vi "Main.vi"(11 "Module Admin":refnum<class "Delacor_lib_QMH_Cloneable Module Admin.lvclass">) -> ()   [LabVIEW 2025, in "Power Supply.lvlib"]
doc: "This template is based off of the Queued Message Handler design pattern and the Queued Message Handler project template that ships with LabVIEW.\n\nThe main difference is that the queue is private to this module and communication between modules is performed via Broadcast and Request events.\n\nRequest events are wrapped in public API methods and are handled in the Event Handling Loop (EHL) of this VI. Any module can register for Broadcast events sent by this module. The EHL generates messages based on user interface actions.\n\nThe Message Handling Loop (MHL) processes messages generated by the EHL, or by other messages. The messages are string values, so new messages can be added easily to the Message Cases case structure in the MHL. Each message cluster can also provide an optional value for Message Data, which is a variant that can be converted to whatever message-specific data is required.\n_____\nBased on DQMH Dev Tools: Project Template 7.1.2.1547."
uses:
  Power Supply.lvlib
  <vilib>/Delacor/Delacor QMH/Libraries/Message Queue_class/Delacor_lib_QMH_Message Queue.lvclass/Delacor_lib_QMH_Message Queue.ctl
  <vilib>/Delacor/Delacor QMH/Libraries/Cloneable Module Admin_class/Delacor_lib_QMH_Cloneable Module Admin.lvclass/Delacor_lib_QMH_Cloneable Module Admin.ctl
  <vilib>/Delacor/Delacor QMH/Libraries/Module Admin_class/Delacor_lib_QMH_Module Admin.lvclass/Delacor_lib_QMH_Module Admin.ctl
  <vilib>/Delacor/Delacor QMH/Libraries/Message Queue_class/Delacor_lib_QMH_Message Queue.lvclass
  Module Data--cluster.ctl
  <vilib>/Utility/miscctls.llb/LVPointTypeDef.ctl
  <vilib>/Delacor/Delacor QMH/Libraries/Message Queue_class/Delacor_lib_QMH_Enqueue Message (Single).vi
  Stop Argument--cluster.ctl
  <vilib>/Delacor/Delacor QMH/Libraries/Cloneable Module Admin_class/Delacor_lib_QMH_Cloneable Module Admin.lvclass
  select child (Reply Payload)--cluster.ctl
  Classes/hardware-selection.ctl
  select child Argument--cluster.ctl
  Classes/generic-power-supply/generic-power-supply.lvclass
  Classes/PSP-603/PSP-603.lvclass
  read config (Reply Payload)--cluster.ctl
  read config Argument--cluster.ctl
  init device (Reply Payload)--cluster.ctl
  init device Argument--cluster.ctl
  close (Reply Payload)--cluster.ctl
  close Argument--cluster.ctl
  output (Reply Payload)--cluster.ctl
  output Argument--cluster.ctl
  set voltage (Reply Payload)--cluster.ctl
  set voltage Argument--cluster.ctl
  set current (Reply Payload)--cluster.ctl
  set current Argument--cluster.ctl
  Controls/Numeric Current.ctl
  read current (Reply Payload)--cluster.ctl
  read current Argument--cluster.ctl
  Controls/Numeric Voltage.ctl
  read voltage (Reply Payload)--cluster.ctl
  read voltage Argument--cluster.ctl
  C:/Users/grove/Desktop/LabVIEW/Git/dqmh-lvoop-template/Libraries/Power Supply/Classes/generic-power-supply/generic-power-supply.lvclass
  C:/Users/grove/Desktop/LabVIEW/Git/dqmh-lvoop-template/Libraries/Power Supply/Classes/PSP-603/PSP-603.lvclass
panel:
  out "error out":errorcluster
  out "Status":string
  in  "Simulate EHL Error":bool
  in  "Simulate MHL Error":bool
  # "Other processes communicate with this Module via its Public API (wrappers for its Request Events).\n\nThis Module communicates with other processes via its Broadcast Events.\nAny process that wants to receive these messages can register for this module's Broadcast events."
  # "This template is for the DQMH framework. See the block diagram for more information on how to use this template."
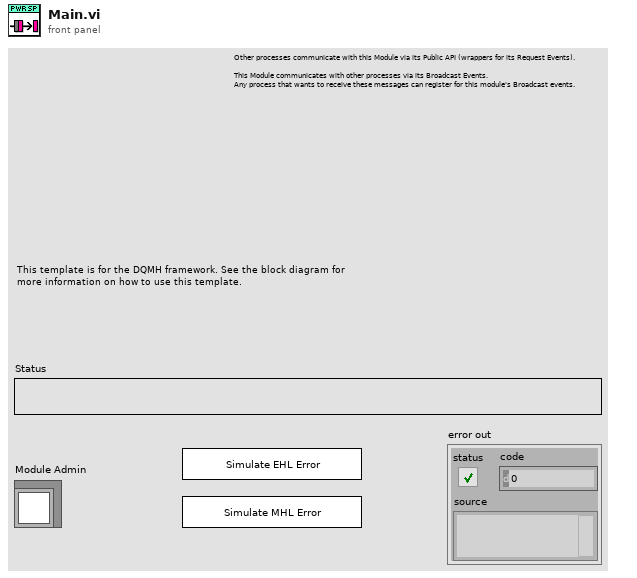
[diagram p1: front panel]
types:
  T1 = typedef "Power Supply.lvlib/Request Events--cluster.ctl" = cluster{"Stop Module":refnum<user-event>, "Show Panel":refnum<user-event>, "Hide Panel":refnum<user-event>, "Show Diagram":refnum<user-event>, "Get Module Execution Status":refnum<user-event>, "select child":refnum<user-event>, "read config":refnum<user-event>, "init device":refnum<user-event>, "close":refnum<user-event>, "output":refnum<user-event>, "set voltage":refnum<user-event>, "set current":refnum<user-event>, "read current":refnum<user-event>, "read voltage":refnum<user-event>}
  T2 = typedef "Power Supply.lvlib/Module Data--cluster.ctl" = cluster{"Status":string, "Power Supply Object":refnum<class "generic-power-supply.lvclass">}
  T3 = enum32{"invalid lock state", "Not Locked", "Locked (No Password)", "Password-protected"}
  T4 = typedef "Power Supply.lvlib/Stop Argument--cluster.ctl" = cluster{"Module ID":i32, "Origin":string, "Exit via Stop Module Req?":bool, "Wait for Module to stop?":bool}
  T5 = typedef "Power Supply.lvlib/select child Argument--cluster.ctl" = cluster{"Module ID":i32, "Enum":T6, "Wait Notifier":refnum<notifier>, "wait for reply":bool}
  T6 = typedef "hardware-selection.ctl" = enum16{"Parent", "Simulation", "PSP-603"}
  T7 = typedef "Power Supply.lvlib/read config Argument--cluster.ctl" = cluster{"Module ID":i32, "config json file":path, "Wait Notifier":refnum<notifier>, "wait for reply":bool}
  T8 = typedef "Power Supply.lvlib/init device Argument--cluster.ctl" = cluster{"Module ID":i32, "Variant":variant, "Wait Notifier":refnum<notifier>, "wait for reply":bool}
  T9 = typedef "Power Supply.lvlib/close Argument--cluster.ctl" = cluster{"Module ID":i32, "Wait Notifier":refnum<notifier>, "wait for reply":bool}
  T10 = typedef "Power Supply.lvlib/output Argument--cluster.ctl" = cluster{"Module ID":i32, "Output On/Off":bool, "Wait Notifier":refnum<notifier>, "wait for reply":bool}
  T11 = typedef "Power Supply.lvlib/set voltage Argument--cluster.ctl" = cluster{"Module ID":i32, "Output Voltage":dbl, "Wait Notifier":refnum<notifier>, "wait for reply":bool}
  T12 = typedef "Power Supply.lvlib/set current Argument--cluster.ctl" = cluster{"Module ID":i32, "Output Current":dbl, "Wait Notifier":refnum<notifier>, "wait for reply":bool}
  T13 = typedef "Power Supply.lvlib/read current Argument--cluster.ctl" = cluster{"Module ID":i32, "Wait Notifier":refnum<notifier>, "wait for reply":bool}
  T14 = typedef "Power Supply.lvlib/read voltage Argument--cluster.ctl" = cluster{"Module ID":i32, "Wait Notifier":refnum<notifier>, "wait for reply":bool}
  T15 = typedef "LVPointTypeDef.ctl" = cluster{"Horizontal":i16, "Vertical":i16}
  T16 = enum32{"Invalid", "Standard", "Closed", "Hidden", "Minimized", "Maximized"}
  T17 = typedef "Power Supply.lvlib/select child (Reply Payload)--cluster.ctl" = cluster{"Module ID":i32, "error":errorcluster}
  T18 = typedef "Power Supply.lvlib/read config (Reply Payload)--cluster.ctl" = cluster{"Module ID":i32, "error":errorcluster}
  T19 = typedef "Power Supply.lvlib/init device (Reply Payload)--cluster.ctl" = cluster{"Module ID":i32, "error":errorcluster}
  T20 = typedef "Power Supply.lvlib/close (Reply Payload)--cluster.ctl" = cluster{"Module ID":i32, "error":errorcluster}
  T21 = typedef "Power Supply.lvlib/output (Reply Payload)--cluster.ctl" = cluster{"Module ID":i32, "error":errorcluster}
  T22 = typedef "Power Supply.lvlib/set voltage (Reply Payload)--cluster.ctl" = cluster{"Module ID":i32, "error":errorcluster}
  T23 = typedef "Power Supply.lvlib/set current (Reply Payload)--cluster.ctl" = cluster{"Module ID":i32, "error":errorcluster}
  T24 = typedef "Power Supply.lvlib/read current (Reply Payload)--cluster.ctl" = cluster{"Module ID":i32, "Amps":T25, "error":errorcluster}
  T25 = typedef "Numeric Current.ctl" = dbl
  T26 = typedef "Power Supply.lvlib/read voltage (Reply Payload)--cluster.ctl" = cluster{"Module ID":i32, "Volts":T27, "error":errorcluster}
  T27 = typedef "Numeric Voltage.ctl" = dbl
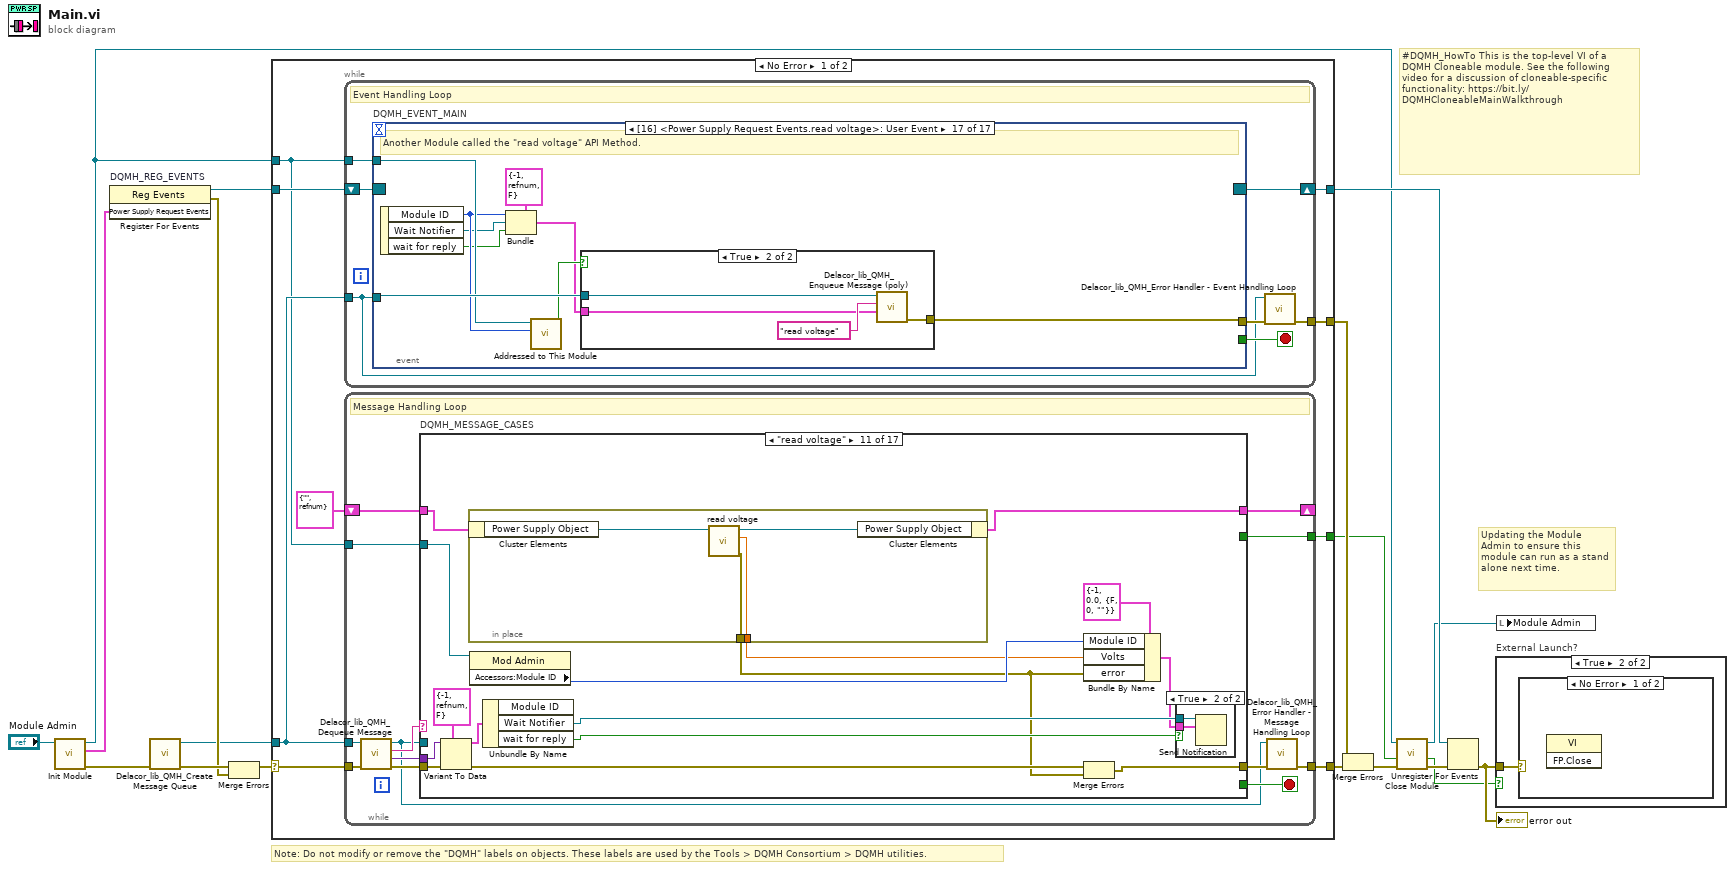
[diagram p0: block diagram]
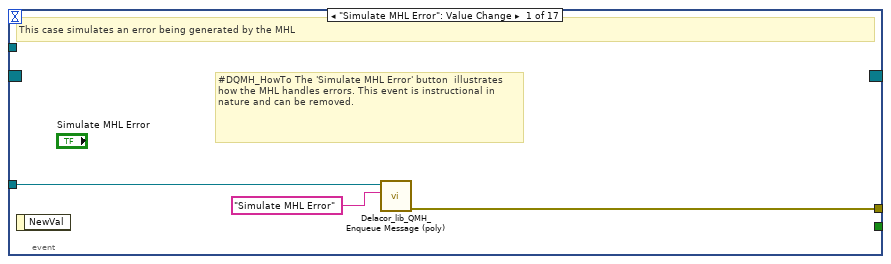
[diagram p2: hidden frame]
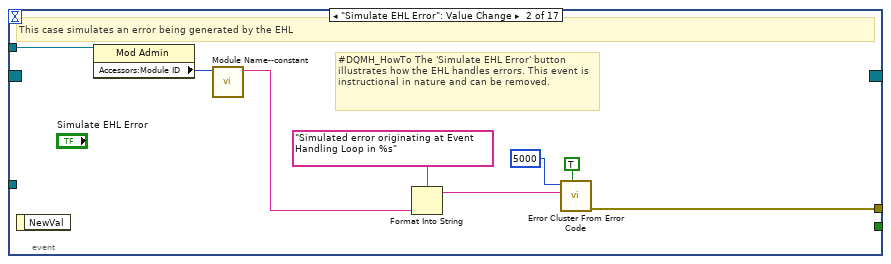
[diagram p3: hidden frame]
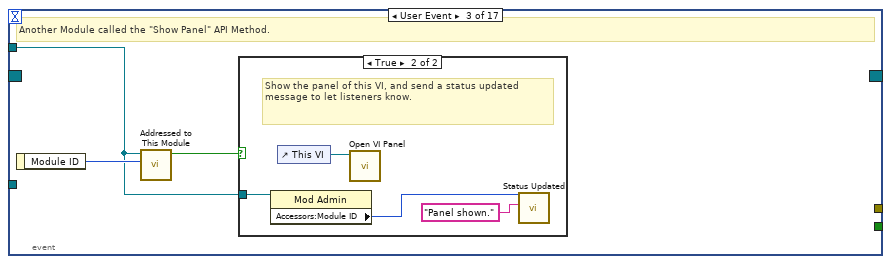
[diagram p4: hidden frame]
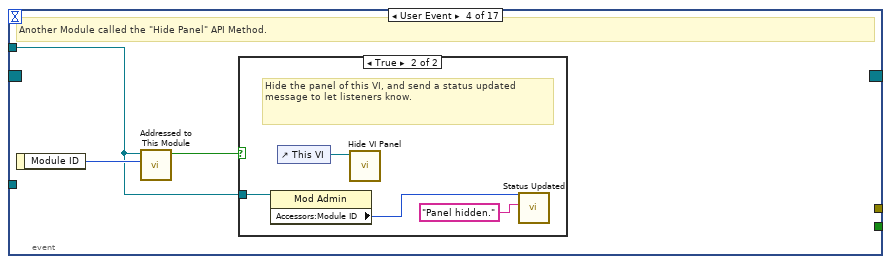
[diagram p6: hidden frame]
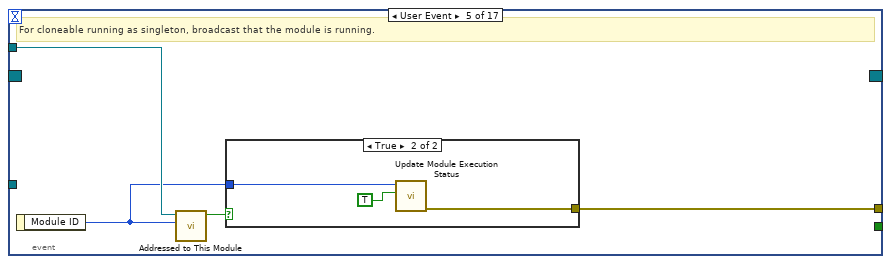
[diagram p8: hidden frame]
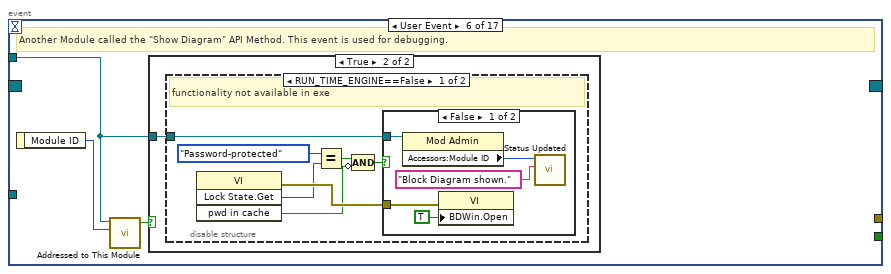
[diagram p10: hidden frame]
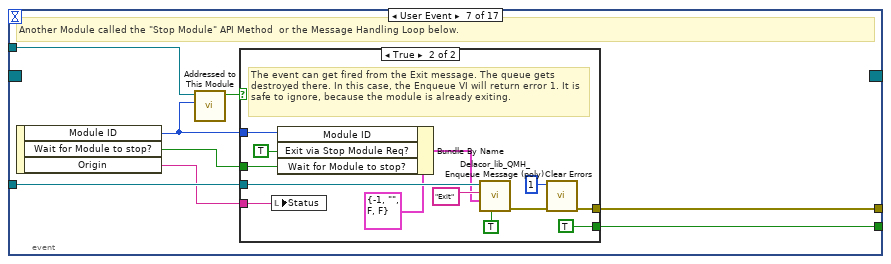
[diagram p14: hidden frame]
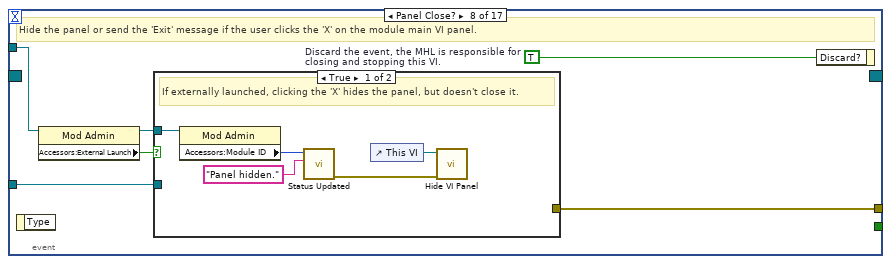
[diagram p16: hidden frame]
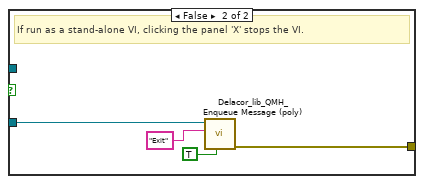
[diagram p17: hidden frame]
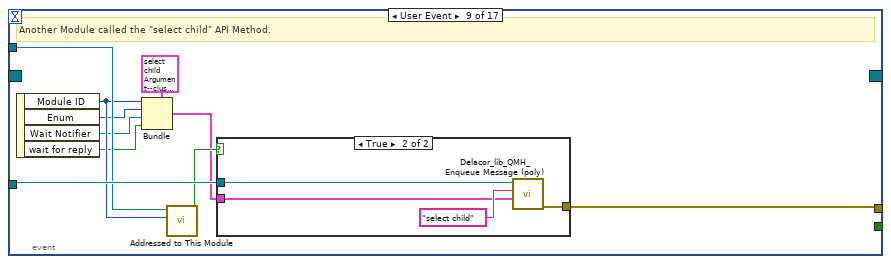
[diagram p18: hidden frame]
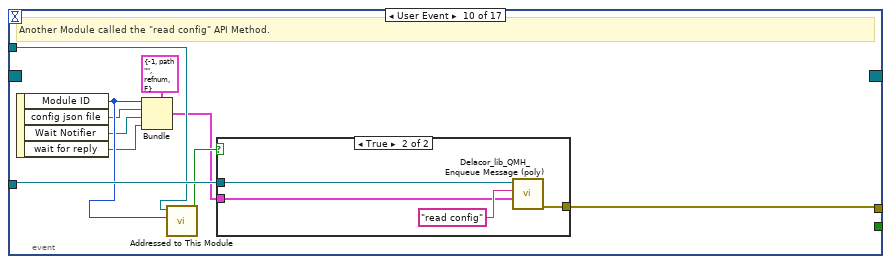
[diagram p20: hidden frame]
diagram:
  # "#DQMH_HowTo This is the top-level VI of a DQMH Cloneable module. See the following video for a discussion of cloneable-specific functionality: https://bit.ly/DQMHCloneableMainWalkthrough"
  # "Note: Do not modify or remove the \"DQMH\" labels on objects. These labels are used by the Tools > DQMH Consortium > DQMH utilities."
  # "Updating the Module Admin to ensure this module can run as a stand alone next time."
  n1 = call "Init Module.vi"("Cloneable Module Admin in"="Module Admin") -> ("error out"=w15:errorcluster, "Power Supply Request Events"=w7:T1, "Cloneable Module Admin out"=w4:refnum<class "Delacor_lib_QMH_Cloneable Module Admin.lvclass">)  [unwired: 8 in]
  n2 = register-events "DQMH_REG_EVENTS"(w7) -> (reference out=w8:refnum<event-registration>, error out=w10:errorcluster)  [unwired: 2 in]
  n3 = call <vilib>:"Delacor_lib_QMH_Create Message Queue.vi"("error in"=w15) -> ("error out"=w12:errorcluster, "Message Queue"=w6:refnum<class "Delacor_lib_QMH_Message Queue.lvclass">)  [unwired: 9 in]
  n4 = Merge Errors(w12, w10) -> (w11:errorcluster)
  n5 = case shown="No Error" w11 {
    selector: w11 -> [w25 w547]
    tunnel: [w27 w546] -> w16
    tunnel: [w24 w545] -> w9
    tunnel: w8 -> [w22 w545]
    tunnel: w6 -> [w21 w538]
    tunnel: [w26 _] -> w17
    tunnel: w4 -> [w20 w541]
    tunnel: [w19 _] -> w2
    frame No Error {
      n6 = while {
        tunnel: w21 -> [w28]
        shift-right: [w31] -> w24
        shift-left: w22 -> [w32]
        tunnel: [w33] -> w26
        tunnel: w20 -> [w29]
        stop <- w30 stop-if-true
        # "Event Handling Loop"
        n7 = event "DQMH_EVENT_MAIN" shown="[16] <Power Supply Request Events.read voltage>: User Event" {
          selector: w32 -> [_ _ _ _ _ _ _ _ _ _ _ _ _ _ _ _ _]
          dyn-events: [_ _ _ _ _ _ _ _ _ _ _ _ _ _ _ _ _] -> w31
          timeout: _ -> [_ _ _ _ _ _ _ _ _ _ _ _ _ _ _ _ _]
          tunnel: [_ _ _ _ _ _ w86 _ _ _ _ _ _ _ _ _ _] -> w30
          tunnel: w28 -> [w36 _ _ _ _ _ w89 w106 w128 w142 w156 w169 w183 w197 w211 w224 w237]
          tunnel: [w37 w45 _ _ w63 _ w90 w109 w119 w133 w147 w161 w174 w188 w202 w216 w229] -> w34
          tunnel: w29 -> [_ w44 w46 w53 w61 w67 w88 w107 w126 w140 w154 w167 w181 w195 w209 w222 w235]
          event "Simulate MHL Error": Value Change {
            # "#DQMH_HowTo The 'Simulate MHL Error' button  illustrates how the MHL handles errors. This event is instructional in nature and can be removed."
            # "This case simulates an error being generated by the MHL"
            n8 = event-data() -> ()  [unwired: 1 in, 1 out]
            n9 = call-poly <vilib>:"Delacor_lib_QMH_Enqueue Message (poly).vi"("Message"="Simulate MHL Error", "Message Queue in"=w36) -> ("error out"=w37:errorcluster)  [unwired: 8 in, 1 out]
          }
          event "Simulate EHL Error": Value Change {
            # "#DQMH_HowTo The 'Simulate EHL Error' button  illustrates how the EHL handles errors. This event is instructional in nature and can be removed."
            # "This case simulates an error being generated by the EHL"
            n10 = event-data() -> ()  [unwired: 1 in, 1 out]
            n11 = property on="Property Node" class="Mod Admin"(reference=w44) -> ("Accessors:Module ID"=w43:i32)  [unwired: 1 in, 2 out]
            n12 = call "Module Name--constant.vi"("Module ID"=w43) -> ("Module Name"=w38:string)  [unwired: 10 in]
            n13 = Format Into String(format string="Simulated error originating at Event Handling Loop in %s", w38) -> (resulting string=w41:string)  [unwired: 2 in, 1 out]
            n14 = call <vilib>:"Error Cluster From Error Code.vi"("show call chain? (False)"=TRUE, "error message (\"\")"=w41, "error code (0)"=5000) -> ("error out"=w45:errorcluster)  [unwired: 6 in]
          }
          event User Event {
            # "Another Module called the \"Show Panel\" API Method."
            n15 = event-data() -> ("Module ID"=w47:i32)  [unwired: 1 in]
            n16 = call "Addressed to This Module.vi"("Module ID from Argument"=w47, "Module Admin"=w46) -> ("Addressed to this instance?"=w48:bool)  [unwired: 8 in, 1 out]
            n17 = case shown="True" w48 {
              tunnel: w46 -> [_ w50]
              frame False {
              }
              frame True {
                # "Show the panel of this VI, and send a status updated message to let listeners know."
                n18 = property on="Property Node" class="Mod Admin"(reference=w50) -> ("Accessors:Module ID"=w49:i32)  [unwired: 1 in, 2 out]
                n19 = control-ref of="This VI"() -> (w52:refnum<vi>)
                n20 = call "Open VI Panel.vi"("VI"=w52) -> ()  [unwired: 10 in, 1 out]
                n21 = call "Status Updated.vi"("Status"="Panel shown." ("format string"), "Module ID"=w49) -> ()  [unwired: 9 in, 1 out]
              }
            }
          }
          event User Event {
            # "Another Module called the \"Hide Panel\" API Method."
            n22 = event-data() -> ("Module ID"=w54:i32)  [unwired: 1 in]
            n23 = call "Addressed to This Module.vi"("Module ID from Argument"=w54, "Module Admin"=w53) -> ("Addressed to this instance?"=w55:bool)  [unwired: 8 in, 1 out]
            n24 = case shown="True" w55 {
              tunnel: w53 -> [_ w57]
              frame False {
              }
              frame True {
                # "Hide the panel of this VI, and send a status updated message to let listeners know."
                n25 = property on="Property Node" class="Mod Admin"(reference=w57) -> ("Accessors:Module ID"=w56:i32)  [unwired: 1 in, 2 out]
                n26 = control-ref of="This VI"() -> (w59:refnum<vi>)
                n27 = call "Hide VI Panel.vi"("VI"=w59) -> ()  [unwired: 10 in, 1 out]
                n28 = call "Status Updated.vi"("Status"="Panel hidden." ("format string"), "Module ID"=w56) -> ()  [unwired: 9 in, 1 out]
              }
            }
          }
          event User Event {
            # "For cloneable running as singleton, broadcast that the module is running."
            n29 = event-data() -> ("Module ID"=w60:i32)  [unwired: 1 in]
            n30 = call "Addressed to This Module.vi"("Module ID from Argument"=w60, "Module Admin"=w61) -> ("Addressed to this instance?"=w62:bool)  [unwired: 8 in, 1 out]
            n31 = case shown="True" w62 {
              tunnel: [_ w66] -> w63
              tunnel: w60 -> [_ w65]
              frame False {
              }
              frame True {
                n32 = call "Update Module Execution Status.vi"("Running?"=TRUE, "Module ID"=w65) -> ("error out"=w66:errorcluster)  [unwired: 9 in]
              }
            }
          }
          event User Event {
            # "Another Module called the \"Show Diagram\" API Method. This event is used for debugging."
            n33 = event-data() -> ("Module ID"=w68:i32)  [unwired: 1 in]
            n34 = call "Addressed to This Module.vi"("Module ID from Argument"=w68, "Module Admin"=w67) -> ("Addressed to this instance?"=w69:bool)  [unwired: 8 in, 1 out]
            n35 = case shown="True" w69 {
              tunnel: w67 -> [_ w70]
              frame False {
              }
              frame True {
                n36 = disable-structure shown="RUN_TIME_ENGINE==False" {
                  disable-tunnel: w70 -> [w71 _]
                  frame condition #0 (active) {
                    # "functionality not available in exe"
                    n37 = invoke on="Invoke Node" class="VI" method="Lock State.Get"() -> (error out=w77:errorcluster, "Get Lock State"=w76:T3, "pwd in cache"=w73:bool)  [unwired: 4 in, 1 out]
                    n38 = Equal?(x=T3."Password-protected", y=w76) -> (x = y?=w74:bool)
                    n39 = Compound Arithmetic op=AND(w74, invert w73) -> (w72:bool)
                    n40 = case shown="False" w72 {
                      tunnel: w77 -> [w82 _]
                      tunnel: w71 -> [w79 _]
                      frame False {
                        n41 = property on="Property Node" class="Mod Admin"(reference=w79) -> ("Accessors:Module ID"=w78:i32)  [unwired: 1 in, 2 out]
                        n42 = property on="Property Node" class="VI"(error in=w82, "BDWin.Open"=TRUE ("Block Diagram Window:Open")) -> ()  [unwired: 1 in, 2 out]
                        n43 = call "Status Updated.vi"("Status"="Block Diagram shown." ("format string"), "Module ID"=w78) -> ()  [unwired: 9 in, 1 out]
                      }
                      frame True {
                        # "Password-protected VI, and the password is not in the cache. Do not show the diagram."
                      }
                    }
                  }
                  frame condition #1 {
                  }
                }
              }
            }
          }
          event User Event {
            # "Another Module called the \"Stop Module\" API Method  or the Message Handling Loop below."
            n44 = event-data() -> ("Module ID"=w84:i32, "Wait for Module to stop?"=w85:bool, "Origin"=w83:string)  [unwired: 1 in]
            n45 = call "Addressed to This Module.vi"("Module ID from Argument"=w84, "Module Admin"=w88) -> ("Addressed to this instance?"=w87:bool)  [unwired: 8 in, 1 out]
            n46 = case shown="True" w87 {
              tunnel: [_ w102] -> w90
              tunnel: w89 -> [_ w98]
              tunnel: [_ TRUE] -> w86
              tunnel: w85 -> [_ w93]
              tunnel: w84 -> [_ w95]
              tunnel: w83 -> [_ w91]
              frame False {
              }
              frame True {
                # "The event can get fired from the Exit message. The queue gets destroyed there. In this case, the Enqueue VI will return error 1. It is safe to ignore, because the module is already exiting."
                n47 = local write "Status"(w91) -> ()
                n48 = Bundle By Name(cluster=T4 {"Module ID"=-1, "Origin"="", "Exit via Stop Module Req?"=FALSE, "Wait for Module to stop?"=FALSE} ("Stop Argument"), "Module ID"=w95, "Exit via Stop Module Req?"=TRUE, "Wait for Module to stop?"=w93) -> (w92:T4)
                n49 = call-poly <vilib>:"Delacor_lib_QMH_Enqueue Message (poly).vi"("Priority Message? (F)"=TRUE, "Message Data"=w92, "Message"="Exit", "Message Queue in"=w98) -> ("error out"=w103:errorcluster)  [unwired: 6 in, 1 out]
                n50 = call <vilib>:"Clear Errors.vi"("error in (no error)"=w103, "specific error code to clear (0: all)"=1) -> ("error out"=w102:errorcluster)  [unwired: 4 in, 1 out]
              }
            }
          }
          event Panel Close? {
            w108 = TRUE  # Discard the event, the MHL is responsible for closing and stopping this VI.
            # "Hide the panel or send the 'Exit' message if the user clicks the 'X' on the module main VI panel."
            n51 = event-data() -> ()  [unwired: 1 in, 1 out]
            n52 = property on="Property Node" class="Mod Admin"(reference=w107) -> (reference out=w104:refnum<class "Delacor_lib_QMH_Cloneable Module Admin.lvclass">, "Accessors:External Launch"=w105:bool)  [unwired: 1 in, 1 out]
            n53 = case shown="True" w105 {
              tunnel: w106 -> [_ w117]
              tunnel: [_ w118] -> w109
              tunnel: w104 -> [w112 _]
              frame True {
                # "If externally launched, clicking the 'X' hides the panel, but doesn't close it."
                n54 = property on="Property Node" class="Mod Admin"(reference=w112) -> ("Accessors:Module ID"=w111:i32)  [unwired: 1 in, 2 out]
                n55 = call "Status Updated.vi"("Status"="Panel hidden." ("format string"), "Module ID"=w111) -> ("error out"=w110:errorcluster)  [unwired: 9 in]
                n56 = control-ref of="This VI"() -> (w114:refnum<vi>)
                n57 = call "Hide VI Panel.vi"("error in"=w110, "VI"=w114) -> ()  [unwired: 9 in, 1 out]
              }
              frame False {
                # "If run as a stand-alone VI, clicking the panel 'X' stops the VI."
                n58 = call-poly <vilib>:"Delacor_lib_QMH_Enqueue Message (poly).vi"("Priority Message? (F)"=TRUE, "Message"="Exit", "Message Queue in"=w117) -> ("error out"=w118:errorcluster)  [unwired: 7 in, 1 out]
              }
            }
            n59 = event-data ("Event Filter Node")("Discard?"=w108) -> ()  [unwired: 1 in, 1 out]
          }
          event User Event {
            # "Another Module called the \"select child\" API Method."
            n60 = event-data() -> ("Module ID"=w123:i32, "Enum"=w122:T6, "Wait Notifier"=w121:refnum<notifier>, "wait for reply"=w120:bool)  [unwired: 1 in]
            n61 = Bundle(cluster=T5 {"Module ID"=-1, "Enum"=enum."PSP-603", "Wait Notifier"=refnum, "wait for reply"=FALSE} ("select child Argument"), "Module ID"=w123, "Enum"=w122, "Wait Notifier"=w121, "wait for reply"=w120) -> (w124:T5)
            n62 = call "Addressed to This Module.vi"("Module ID from Argument"=w123, "Module Admin"=w126) -> ("Addressed to this instance?"=w127:bool)  [unwired: 8 in, 1 out]
            n63 = case shown="True" w127 {
              tunnel: w128 -> [_ w132]
              tunnel: w124 -> [_ w130]
              tunnel: [_ w129] -> w119
              frame False {
              }
              frame True {
                n64 = call-poly <vilib>:"Delacor_lib_QMH_Enqueue Message (poly).vi"("Message Data"=w130, "Message"="select child", "Message Queue in"=w132) -> ("error out"=w129:errorcluster)  [unwired: 7 in, 1 out]
              }
            }
          }
          event User Event {
            # "Another Module called the \"read config\" API Method."
            n65 = event-data() -> ("Module ID"=w137:i32, "config json file"=w136:path, "Wait Notifier"=w135:refnum<notifier>, "wait for reply"=w134:bool)  [unwired: 1 in]
            n66 = Bundle(cluster=T7 {"Module ID"=-1, "config json file"=path "", "Wait Notifier"=refnum, "wait for reply"=FALSE} ("read config Argument"), "Module ID"=w137, "config json file"=w136, "Wait Notifier"=w135, "wait for reply"=w134) -> (w138:T7)
            n67 = call "Addressed to This Module.vi"("Module ID from Argument"=w137, "Module Admin"=w140) -> ("Addressed to this instance?"=w141:bool)  [unwired: 8 in, 1 out]
            n68 = case shown="True" w141 {
              tunnel: w142 -> [_ w146]
              tunnel: w138 -> [_ w144]
              tunnel: [_ w143] -> w133
              frame False {
              }
              frame True {
                n69 = call-poly <vilib>:"Delacor_lib_QMH_Enqueue Message (poly).vi"("Message Data"=w144, "Message"="read config", "Message Queue in"=w146) -> ("error out"=w143:errorcluster)  [unwired: 7 in, 1 out]
              }
            }
          }
          event User Event {
            # "Another Module called the \"init device\" API Method."
            n70 = event-data() -> ("Module ID"=w151:i32, "Variant"=w150:variant, "Wait Notifier"=w149:refnum<notifier>, "wait for reply"=w148:bool)  [unwired: 1 in]
            n71 = Bundle(cluster=T8 {"Module ID"=-1, "Variant"=variant, "Wait Notifier"=refnum, "wait for reply"=FALSE} ("init device Argument"), "Module ID"=w151, "Variant"=w150, "Wait Notifier"=w149, "wait for reply"=w148) -> (w152:T8)
            n72 = call "Addressed to This Module.vi"("Module ID from Argument"=w151, "Module Admin"=w154) -> ("Addressed to this instance?"=w155:bool)  [unwired: 8 in, 1 out]
            n73 = case shown="True" w155 {
              tunnel: w156 -> [_ w160]
              tunnel: w152 -> [_ w158]
              tunnel: [_ w157] -> w147
              frame False {
              }
              frame True {
                n74 = call-poly <vilib>:"Delacor_lib_QMH_Enqueue Message (poly).vi"("Message Data"=w158, "Message"="init device", "Message Queue in"=w160) -> ("error out"=w157:errorcluster)  [unwired: 7 in, 1 out]
              }
            }
          }
          event User Event {
            # "Another Module called the \"close\" API Method."
            n75 = event-data() -> ("Module ID"=w164:i32, "Wait Notifier"=w163:refnum<notifier>, "wait for reply"=w162:bool)  [unwired: 1 in]
            n76 = Bundle(cluster=T9 {"Module ID"=-1, "Wait Notifier"=refnum, "wait for reply"=FALSE} ("close Argument"), "Module ID"=w164, "Wait Notifier"=w163, "wait for reply"=w162) -> (w165:T9)
            n77 = call "Addressed to This Module.vi"("Module ID from Argument"=w164, "Module Admin"=w167) -> ("Addressed to this instance?"=w168:bool)  [unwired: 8 in, 1 out]
            n78 = case shown="True" w168 {
              tunnel: w169 -> [_ w173]
              tunnel: w165 -> [_ w171]
              tunnel: [_ w170] -> w161
              frame False {
              }
              frame True {
                n79 = call-poly <vilib>:"Delacor_lib_QMH_Enqueue Message (poly).vi"("Message Data"=w171, "Message"="close", "Message Queue in"=w173) -> ("error out"=w170:errorcluster)  [unwired: 7 in, 1 out]
              }
            }
          }
          event User Event {
            # "Another Module called the \"output\" API Method."
            n80 = event-data() -> ("Module ID"=w178:i32, "Output On/Off"=w177:bool, "Wait Notifier"=w176:refnum<notifier>, "wait for reply"=w175:bool)  [unwired: 1 in]
            n81 = Bundle(cluster=T10 {"Module ID"=-1, "Output On/Off"=FALSE, "Wait Notifier"=refnum, "wait for reply"=FALSE} ("output Argument"), "Module ID"=w178, "Output On/Off"=w177, "Wait Notifier"=w176, "wait for reply"=w175) -> (w179:T10)
            n82 = call "Addressed to This Module.vi"("Module ID from Argument"=w178, "Module Admin"=w181) -> ("Addressed to this instance?"=w182:bool)  [unwired: 8 in, 1 out]
            n83 = case shown="True" w182 {
              tunnel: w183 -> [_ w187]
              tunnel: w179 -> [_ w185]
              tunnel: [_ w184] -> w174
              frame False {
              }
              frame True {
                n84 = call-poly <vilib>:"Delacor_lib_QMH_Enqueue Message (poly).vi"("Message Data"=w185, "Message"="output", "Message Queue in"=w187) -> ("error out"=w184:errorcluster)  [unwired: 7 in, 1 out]
              }
            }
          }
          event User Event {
            # "Another Module called the \"set voltage\" API Method."
            n85 = event-data() -> ("Module ID"=w192:i32, "Output Voltage"=w191:dbl, "Wait Notifier"=w190:refnum<notifier>, "wait for reply"=w189:bool)  [unwired: 1 in]
            n86 = Bundle(cluster=T11 {"Module ID"=-1, "Output Voltage"=10.0, "Wait Notifier"=refnum, "wait for reply"=FALSE} ("set voltage Argument"), "Module ID"=w192, "Output Voltage"=w191, "Wait Notifier"=w190, "wait for reply"=w189) -> (w193:T11)
            n87 = call "Addressed to This Module.vi"("Module ID from Argument"=w192, "Module Admin"=w195) -> ("Addressed to this instance?"=w196:bool)  [unwired: 8 in, 1 out]
            n88 = case shown="True" w196 {
              tunnel: w197 -> [_ w201]
              tunnel: w193 -> [_ w199]
              tunnel: [_ w198] -> w188
              frame False {
              }
              frame True {
                n89 = call-poly <vilib>:"Delacor_lib_QMH_Enqueue Message (poly).vi"("Message Data"=w199, "Message"="set voltage", "Message Queue in"=w201) -> ("error out"=w198:errorcluster)  [unwired: 7 in, 1 out]
              }
            }
          }
          event User Event {
            # "Another Module called the \"set current\" API Method."
            n90 = event-data() -> ("Module ID"=w206:i32, "Output Current"=w205:dbl, "Wait Notifier"=w204:refnum<notifier>, "wait for reply"=w203:bool)  [unwired: 1 in]
            n91 = Bundle(cluster=T12 {"Module ID"=-1, "Output Current"=0.05, "Wait Notifier"=refnum, "wait for reply"=FALSE} ("set current Argument"), "Module ID"=w206, "Output Current"=w205, "Wait Notifier"=w204, "wait for reply"=w203) -> (w207:T12)
            n92 = call "Addressed to This Module.vi"("Module ID from Argument"=w206, "Module Admin"=w209) -> ("Addressed to this instance?"=w210:bool)  [unwired: 8 in, 1 out]
            n93 = case shown="True" w210 {
              tunnel: w211 -> [_ w215]
              tunnel: w207 -> [_ w213]
              tunnel: [_ w212] -> w202
              frame False {
              }
              frame True {
                n94 = call-poly <vilib>:"Delacor_lib_QMH_Enqueue Message (poly).vi"("Message Data"=w213, "Message"="set current", "Message Queue in"=w215) -> ("error out"=w212:errorcluster)  [unwired: 7 in, 1 out]
              }
            }
          }
          event User Event {
            # "Another Module called the \"read current\" API Method."
            n95 = event-data() -> ("Module ID"=w219:i32, "Wait Notifier"=w218:refnum<notifier>, "wait for reply"=w217:bool)  [unwired: 1 in]
            n96 = Bundle(cluster=T13 {"Module ID"=-1, "Wait Notifier"=refnum, "wait for reply"=FALSE} ("read current Argument"), "Module ID"=w219, "Wait Notifier"=w218, "wait for reply"=w217) -> (w220:T13)
            n97 = call "Addressed to This Module.vi"("Module ID from Argument"=w219, "Module Admin"=w222) -> ("Addressed to this instance?"=w223:bool)  [unwired: 8 in, 1 out]
            n98 = case shown="True" w223 {
              tunnel: w224 -> [_ w228]
              tunnel: w220 -> [_ w226]
              tunnel: [_ w225] -> w216
              frame False {
              }
              frame True {
                n99 = call-poly <vilib>:"Delacor_lib_QMH_Enqueue Message (poly).vi"("Message Data"=w226, "Message"="read current", "Message Queue in"=w228) -> ("error out"=w225:errorcluster)  [unwired: 7 in, 1 out]
              }
            }
          }
          event User Event {
            # "Another Module called the \"read voltage\" API Method."
            n100 = event-data() -> ("Module ID"=w232:i32, "Wait Notifier"=w231:refnum<notifier>, "wait for reply"=w230:bool)  [unwired: 1 in]
            n101 = Bundle(cluster=T14 {"Module ID"=-1, "Wait Notifier"=refnum, "wait for reply"=FALSE} ("read voltage Argument"), "Module ID"=w232, "Wait Notifier"=w231, "wait for reply"=w230) -> (w233:T14)
            n102 = call "Addressed to This Module.vi"("Module ID from Argument"=w232, "Module Admin"=w235) -> ("Addressed to this instance?"=w236:bool)  [unwired: 8 in, 1 out]
            n103 = case shown="True" w236 {
              tunnel: w237 -> [_ w241]
              tunnel: w233 -> [_ w239]
              tunnel: [_ w238] -> w229
              frame False {
              }
              frame True {
                n104 = call-poly <vilib>:"Delacor_lib_QMH_Enqueue Message (poly).vi"("Message Data"=w239, "Message"="read voltage", "Message Queue in"=w241) -> ("error out"=w238:errorcluster)  [unwired: 7 in, 1 out]
              }
            }
          }
        }
        n105 = call-dynamic "Delacor_lib_QMH_Error Handler - Event Handling Loop.vi"("error in"=w34, "Message Queue in"=w28) -> ("dup error in"=w33:errorcluster)  [unwired: 8 in, 1 out]
      }
      n106 = while {
        tunnel: w21 -> [w242]
        shift-right: [w249] -> _
        shift-left: T2 {"Status"="", "Power Supply Object"=refnum} ("Data Cluster") -> [w250]
        tunnel: w25 -> [w253]
        tunnel: [w251] -> w27
        tunnel: w20 -> [w244]
        tunnel: [w243] -> w19
        stop <- w248 stop-if-true
        # "Message Handling Loop"
        n107 = call-dynamic "Delacor_lib_QMH_Dequeue Message.vi"("error in"=w253, "Message Queue in"=w242) -> ("error out"=w252:errorcluster, "Message Data"=w246:variant, "Message"=w247:string, "Message Queue out"=w245:refnum<class "Delacor_lib_QMH_Message Queue.lvclass">)  [unwired: 6 in]
        n108 = case "DQMH_MESSAGE_CASES" shown="\"read voltage\"" w247 {
          selector: w247 -> [_ _ _ _ _ _ _ _ _ _ _ _ _ _ _ _ w527]
          tunnel: w245 -> [_ _ _ _ _ _ _ _ _ _ _ _ _ w482 _ w519 _]
          tunnel: w252 -> [w273 w277 w293 w316 w338 w359 w380 w402 w424 w446 w468 w477 w479 w491 w508 w525 w536]
          tunnel: [w271 w277 w284 w307 w329 w350 w371 w393 w415 w437 w459 w476 w479 w487 w507 w520 w537] -> w254
          tunnel: w250 -> [w264 w276 w281 w304 w326 w347 w368 w390 w412 w434 w456 w475 w478 w486 w505 w518 w534]
          tunnel: [w263 w276 w280 w303 w325 w346 w367 w389 w411 w433 w455 w475 w478 w486 w505 w518 w534] -> w249
          tunnel: [_ _ _ _ _ _ _ _ _ _ _ _ _ _ _ w517 _] -> w248
          tunnel: w246 -> [_ _ w291 w314 w336 w357 w378 w400 w422 w444 w466 _ _ w485 _ w515 _]
          tunnel: w244 -> [w259 _ w282 w305 w327 w348 w369 w391 w413 w435 w457 _ _ w484 w503 w510 w533]
          tunnel: [_ _ _ _ _ _ _ _ _ _ _ _ _ _ _ w513 _] -> w243
          frame "Initialize" {
            w256 = "Initial Message" ("Initial Message")
            # "#DQMH_CodeNeeded - Initialize the appearance of the front panel."
            # "#DQMH_CodeNeeded - Initialize your state data here."
            # "Initialize - Any operation that needs to be done before the module can receive messages. Synchronize Caller Events.vi will inform Start Module.vi that the module has launched and is ready to receive messages. Module Did Init.vi will broadcast that the module initialized."
            n109 = call "Synchronize Caller Events.vi"("error in"=w273, "Module Admin"=w259) -> ("error out"=w272:errorcluster, "Module Admin out"=w258:refnum<class "Delacor_lib_QMH_Cloneable Module Admin.lvclass">)  [unwired: 8 in]
            n110 = property on="Property Node" class="Mod Admin"(reference=w258) -> ("Accessors:Module ID"=w255:i32, "Accessors:External Launch"=w260:bool)  [unwired: 1 in, 2 out]
            n111 = call "Module Name--constant.vi"("Module ID"=w255) -> ("Module Name"=w268:string)  [unwired: 10 in]
            n112 = property on="Property Node" class="VI"("Front Panel.Title"=w268) -> (reference out=w270:refnum<vi>, error out=w275:errorcluster)  [unwired: 2 in]
            n113 = Select(t=T16."Hidden" ("State"), s=w260, f=T16."Standard" ("State")) -> (s? t:f=w265:T16)
            n114 = invoke on="Invoke Node" class="VI" method="FP.Open"(reference=w270, error in=w275, "State"=w265) -> (reference out=w269:refnum<vi>, error out=w274:errorcluster)  [unwired: 2 in, 3 out]
            n115 = Bundle By Name(cluster=w264, "Status"=w256) -> (w263:T2)
            n116 = invoke on="Invoke Node" class="VI" method="FP.Center"(reference=w269, error in=w274) -> ()  [unwired: 1 in, 3 out]
            n117 = property on="Pane" class="Pane"("Origin"=T15 {"Horizontal"=0, "Vertical"=0}) -> ()  [unwired: 2 in, 2 out]
            n118 = call "Module Name--constant.vi"("Module ID"=w255) -> ("Module Name"=w261:string)  [unwired: 10 in]
            n119 = call "Module Did Init.vi"("error in"=w272, "Initialized?"=TRUE, "Origin"=w261, "Module ID"=w255) -> ("error out"=w271:errorcluster)  [unwired: 7 in]
            "Status" <- w256
          }
          frame "---Module Specific---" {
            # "Separator -- The following cases handle messages specific to this Module."
          }
          frame "select child" {
            w279 = errorcluster {"status"=FALSE, "code"=0, "source"=""} ("error")
            n120 = Variant To Data(error in=w293, type=T5 {"Module ID"=-1, "Enum"=enum."PSP-603", "Wait Notifier"=refnum, "wait for reply"=FALSE} ("select child Argument"), Variant=w291) -> (data=w289:T5, error out=w292:errorcluster)
            n121 = property class="Mod Admin"(reference=w282) -> ("Accessors:Module ID"=w283:i32)  [unwired: 1 in, 2 out]
            n122 = Unbundle By Name(w289) -> ("Enum"=w278:T6, "Wait Notifier"=w288:refnum<notifier>, "wait for reply"=w287:bool)  [unwired: 1 out]
            n123 = in-place {
              in-place-border: w278 -> [w294]
              n124 = in-place-cluster #1(w281) -> ()  [unwired: 1 out]
              n125 = case shown="\"Parent\"" w294 {
                tunnel: [refnum<class "generic-power-supply.lvclass"> refnum ("Power Supply.lvlib:generic-power-supply.lvclass") refnum<class "generic-power-supply.lvclass"> refnum ("Power Supply.lvlib:generic-power-supply.lvclass") refnum<class "PSP-603.lvclass"> refnum ("Power Supply.lvlib:PSP-603.lvclass")] -> w295
                frame "Simulation" {
                }
                frame "Parent" {
                }
                frame "PSP-603" {
                }
              }
              n126 = in-place-cluster #1("Power Supply Object"=w295) -> (w280:T2)
            }
            n127 = Bundle By Name(cluster=T17 {"Module ID"=-1, "error"={"status"=FALSE, "code"=0, "source"=""}} ("select child (Reply Payload)"), "Module ID"=w283, "error"=w279) -> (w286:T17)
            n128 = Merge Errors(w292, w279) -> (w284:errorcluster)
            n129 = case "DQMH_FIRE_NOTIFIER" shown="True" w287 {
              tunnel: w288 -> [_ w300]
              tunnel: w286 -> [_ w299]
              frame False {
              }
              frame True {
                n130 = Send Notification(notification=w299, notifier=w300) -> ()  [unwired: 1 in, 2 out]
              }
            }
          }
          frame "read config" {
            n131 = Variant To Data(error in=w316, type=T7 {"Module ID"=-1, "config json file"=path "", "Wait Notifier"=refnum, "wait for reply"=FALSE} ("read config Argument"), Variant=w314) -> (data=w312:T7, error out=w315:errorcluster)
            n132 = property class="Mod Admin"(reference=w305) -> ("Accessors:Module ID"=w306:i32)  [unwired: 1 in, 2 out]
            n133 = Unbundle By Name(w312) -> ("config json file"=w302:path, "Wait Notifier"=w311:refnum<notifier>, "wait for reply"=w310:bool)  [unwired: 1 out]
            n134 = in-place {
              in-place-border: w302 -> [w318]
              in-place-border: [w317] -> w301
              n135 = in-place-cluster #2(w304) -> ("Power Supply Object"=w320:refnum<class "generic-power-supply.lvclass">)
              n136 = call-dynamic "read config.vi"("File Path"=w318, "generic-power-supply in"=w320) -> ("error out"=w317:errorcluster, "generic-power-supply out"=w319:refnum<class "generic-power-supply.lvclass">)  [unwired: 8 in]
              n137 = in-place-cluster #2("Power Supply Object"=w319) -> (w303:T2)
            }
            n138 = Bundle By Name(cluster=T18 {"Module ID"=-1, "error"={"status"=FALSE, "code"=0, "source"=""}} ("read config (Reply Payload)"), "Module ID"=w306, "error"=w301) -> (w309:T18)
            n139 = Merge Errors(w315, w301) -> (w307:errorcluster)
            n140 = case "DQMH_FIRE_NOTIFIER" shown="True" w310 {
              tunnel: w311 -> [_ w322]
              tunnel: w309 -> [_ w321]
              frame False {
              }
              frame True {
                n141 = Send Notification(notification=w321, notifier=w322) -> ()  [unwired: 1 in, 2 out]
              }
            }
          }
          frame "init device" {
            n142 = Variant To Data(error in=w338, type=T8 {"Module ID"=-1, "Variant"=variant, "Wait Notifier"=refnum, "wait for reply"=FALSE} ("init device Argument"), Variant=w336) -> (data=w334:T8, error out=w337:errorcluster)
            n143 = property class="Mod Admin"(reference=w327) -> ("Accessors:Module ID"=w328:i32)  [unwired: 1 in, 2 out]
            n144 = Unbundle By Name(w334) -> ("Variant"=w323:variant, "Wait Notifier"=w333:refnum<notifier>, "wait for reply"=w332:bool)  [unwired: 1 out]
            n145 = in-place {
              in-place-border: [w340] -> w324
              in-place-border: w323 -> [w339]
              n146 = in-place-cluster #3(w326) -> ("Power Supply Object"=w341:refnum<class "generic-power-supply.lvclass">)
              n147 = call-dynamic "init.vi"("Variant"=w339, "generic-power-supply in"=w341) -> ("error out"=w340:errorcluster, "generic-power-supply out"=w342:refnum<class "generic-power-supply.lvclass">)  [unwired: 8 in]
              n148 = in-place-cluster #3("Power Supply Object"=w342) -> (w325:T2)
            }
            n149 = Bundle By Name(cluster=T19 {"Module ID"=-1, "error"={"status"=FALSE, "code"=0, "source"=""}} ("init device (Reply Payload)"), "Module ID"=w328, "error"=w324) -> (w331:T19)
            n150 = Merge Errors(w337, w324) -> (w329:errorcluster)
            n151 = case "DQMH_FIRE_NOTIFIER" shown="True" w332 {
              tunnel: w333 -> [_ w344]
              tunnel: w331 -> [_ w343]
              frame False {
              }
              frame True {
                n152 = Send Notification(notification=w343, notifier=w344) -> ()  [unwired: 1 in, 2 out]
              }
            }
          }
          frame "close" {
            n153 = Variant To Data(error in=w359, type=T9 {"Module ID"=-1, "Wait Notifier"=refnum, "wait for reply"=FALSE} ("close Argument"), Variant=w357) -> (data=w355:T9, error out=w358:errorcluster)
            n154 = in-place {
              in-place-border: [w360] -> w345
              n155 = in-place-cluster #4(w347) -> ("Power Supply Object"=w362:refnum<class "generic-power-supply.lvclass">)
              n156 = call-dynamic "close.vi"("generic-power-supply in"=w362) -> ("error out"=w360:errorcluster, "generic-power-supply out"=w361:refnum<class "generic-power-supply.lvclass">)  [unwired: 9 in]
              n157 = in-place-cluster #4("Power Supply Object"=w361) -> (w346:T2)
            }
            n158 = property class="Mod Admin"(reference=w348) -> ("Accessors:Module ID"=w349:i32)  [unwired: 1 in, 2 out]
            n159 = Unbundle By Name(w355) -> ("Wait Notifier"=w354:refnum<notifier>, "wait for reply"=w353:bool)  [unwired: 1 out]
            n160 = Bundle By Name(cluster=T20 {"Module ID"=-1, "error"={"status"=FALSE, "code"=0, "source"=""}} ("close (Reply Payload)"), "Module ID"=w349, "error"=w345) -> (w352:T20)
            n161 = Merge Errors(w358, w345) -> (w350:errorcluster)
            n162 = case "DQMH_FIRE_NOTIFIER" shown="True" w353 {
              tunnel: w354 -> [_ w364]
              tunnel: w352 -> [_ w363]
              frame False {
              }
              frame True {
                n163 = Send Notification(notification=w363, notifier=w364) -> ()  [unwired: 1 in, 2 out]
              }
            }
          }
          frame "output" {
            n164 = property class="Mod Admin"(reference=w369) -> ("Accessors:Module ID"=w370:i32)  [unwired: 1 in, 2 out]
            n165 = Variant To Data(error in=w380, type=T10 {"Module ID"=-1, "Output On/Off"=FALSE, "Wait Notifier"=refnum, "wait for reply"=FALSE} ("output Argument"), Variant=w378) -> (data=w376:T10, error out=w379:errorcluster)
            n166 = Unbundle By Name(w376) -> ("Output On/Off"=w366:bool, "Wait Notifier"=w375:refnum<notifier>, "wait for reply"=w374:bool)  [unwired: 1 out]
            n167 = in-place {
              in-place-border: w366 -> [w382]
              in-place-border: [w381] -> w365
              n168 = in-place-cluster #5(w368) -> ("Power Supply Object"=w384:refnum<class "generic-power-supply.lvclass">)
              n169 = call-dynamic "output.vi"("Output [on/off]"=w382, "generic-power-supply in"=w384) -> ("error out"=w381:errorcluster, "generic-power-supply out"=w383:refnum<class "generic-power-supply.lvclass">)  [unwired: 8 in]
              n170 = in-place-cluster #5("Power Supply Object"=w383) -> (w367:T2)
            }
            n171 = Bundle By Name(cluster=T21 {"Module ID"=-1, "error"={"status"=FALSE, "code"=0, "source"=""}} ("output (Reply Payload)"), "Module ID"=w370, "error"=w365) -> (w373:T21)
            n172 = Merge Errors(w379, w365) -> (w371:errorcluster)
            n173 = case "DQMH_FIRE_NOTIFIER" shown="True" w374 {
              tunnel: w375 -> [_ w386]
              tunnel: w373 -> [_ w385]
              frame False {
              }
              frame True {
                n174 = Send Notification(notification=w385, notifier=w386) -> ()  [unwired: 1 in, 2 out]
              }
            }
          }
          frame "set voltage" {
            n175 = Variant To Data(error in=w402, type=T11 {"Module ID"=-1, "Output Voltage"=10.0, "Wait Notifier"=refnum, "wait for reply"=FALSE} ("set voltage Argument"), Variant=w400) -> (data=w398:T11, error out=w401:errorcluster)
            n176 = property class="Mod Admin"(reference=w391) -> ("Accessors:Module ID"=w392:i32)  [unwired: 1 in, 2 out]
            n177 = Unbundle By Name(w398) -> ("Output Voltage"=w388:dbl, "Wait Notifier"=w397:refnum<notifier>, "wait for reply"=w396:bool)  [unwired: 1 out]
            n178 = in-place {
              in-place-border: w388 -> [w404]
              in-place-border: [w403] -> w387
              n179 = in-place-cluster #6(w390) -> ("Power Supply Object"=w406:refnum<class "generic-power-supply.lvclass">)
              n180 = call-dynamic "set voltage.vi"("Voltage"=w404, "generic-power-supply in"=w406) -> ("error out"=w403:errorcluster, "generic-power-supply out"=w405:refnum<class "generic-power-supply.lvclass">)  [unwired: 8 in]
              n181 = in-place-cluster #6("Power Supply Object"=w405) -> (w389:T2)
            }
            n182 = Bundle By Name(cluster=T22 {"Module ID"=-1, "error"={"status"=FALSE, "code"=0, "source"=""}} ("set voltage (Reply Payload)"), "Module ID"=w392, "error"=w387) -> (w395:T22)
            n183 = Merge Errors(w401, w387) -> (w393:errorcluster)
            n184 = case "DQMH_FIRE_NOTIFIER" shown="True" w396 {
              tunnel: w397 -> [_ w408]
              tunnel: w395 -> [_ w407]
              frame False {
              }
              frame True {
                n185 = Send Notification(notification=w407, notifier=w408) -> ()  [unwired: 1 in, 2 out]
              }
            }
          }
          frame "set current" {
            n186 = property class="Mod Admin"(reference=w413) -> ("Accessors:Module ID"=w414:i32)  [unwired: 1 in, 2 out]
            n187 = Variant To Data(error in=w424, type=T12 {"Module ID"=-1, "Output Current"=0.05, "Wait Notifier"=refnum, "wait for reply"=FALSE} ("set current Argument"), Variant=w422) -> (data=w420:T12, error out=w423:errorcluster)
            n188 = Unbundle By Name(w420) -> ("Output Current"=w410:dbl, "Wait Notifier"=w419:refnum<notifier>, "wait for reply"=w418:bool)  [unwired: 1 out]
            n189 = in-place {
              in-place-border: w410 -> [w426]
              in-place-border: [w425] -> w409
              n190 = in-place-cluster #7(w412) -> ("Power Supply Object"=w428:refnum<class "generic-power-supply.lvclass">)
              n191 = call-dynamic "set current.vi"("Current [A]"=w426, "generic-power-supply in"=w428) -> ("error out"=w425:errorcluster, "generic-power-supply out"=w427:refnum<class "generic-power-supply.lvclass">)  [unwired: 8 in]
              n192 = in-place-cluster #7("Power Supply Object"=w427) -> (w411:T2)
            }
            n193 = Bundle By Name(cluster=T23 {"Module ID"=-1, "error"={"status"=FALSE, "code"=0, "source"=""}} ("set current (Reply Payload)"), "Module ID"=w414, "error"=w409) -> (w417:T23)
            n194 = Merge Errors(w423, w409) -> (w415:errorcluster)
            n195 = case "DQMH_FIRE_NOTIFIER" shown="True" w418 {
              tunnel: w419 -> [_ w430]
              tunnel: w417 -> [_ w429]
              frame False {
              }
              frame True {
                n196 = Send Notification(notification=w429, notifier=w430) -> ()  [unwired: 1 in, 2 out]
              }
            }
          }
          frame "read current" {
            n197 = Variant To Data(error in=w446, type=T13 {"Module ID"=-1, "Wait Notifier"=refnum, "wait for reply"=FALSE} ("read current Argument"), Variant=w444) -> (data=w442:T13, error out=w445:errorcluster)
            n198 = property class="Mod Admin"(reference=w435) -> ("Accessors:Module ID"=w436:i32)  [unwired: 1 in, 2 out]
            n199 = in-place {
              in-place-border: [w448] -> w432
              in-place-border: [w447] -> w431
              n200 = in-place-cluster #8(w434) -> ("Power Supply Object"=w450:refnum<class "generic-power-supply.lvclass">)
              n201 = call-dynamic "read current.vi"("generic-power-supply in"=w450) -> ("error out"=w447:errorcluster, "Current [A]"=w448:dbl, "generic-power-supply out"=w449:refnum<class "generic-power-supply.lvclass">)  [unwired: 8 in]
              n202 = in-place-cluster #8("Power Supply Object"=w449) -> (w433:T2)
            }
            n203 = Unbundle By Name(w442) -> ("Wait Notifier"=w441:refnum<notifier>, "wait for reply"=w440:bool)  [unwired: 1 out]
            n204 = Bundle By Name(cluster=T24 {"Module ID"=-1, "Amps"=0.0, "error"={"status"=FALSE, "code"=0, "source"=""}} ("read current (Reply Payload)"), "Module ID"=w436, "Amps"=w432, "error"=w431) -> (w439:T24)
            n205 = Merge Errors(w445, w431) -> (w437:errorcluster)
            n206 = case "DQMH_FIRE_NOTIFIER" shown="True" w440 {
              tunnel: w441 -> [_ w452]
              tunnel: w439 -> [_ w451]
              frame False {
              }
              frame True {
                n207 = Send Notification(notification=w451, notifier=w452) -> ()  [unwired: 1 in, 2 out]
              }
            }
          }
          frame "read voltage" {
            n208 = Variant To Data(error in=w468, type=T14 {"Module ID"=-1, "Wait Notifier"=refnum, "wait for reply"=FALSE} ("read voltage Argument"), Variant=w466) -> (data=w464:T14, error out=w467:errorcluster)
            n209 = in-place {
              in-place-border: [w470] -> w454
              in-place-border: [w469] -> w453
              n210 = in-place-cluster #9(w456) -> ("Power Supply Object"=w472:refnum<class "generic-power-supply.lvclass">)
              n211 = call-dynamic "read voltage.vi"("generic-power-supply in"=w472) -> ("error out"=w469:errorcluster, "Voltage [V]"=w470:dbl, "generic-power-supply out"=w471:refnum<class "generic-power-supply.lvclass">)  [unwired: 8 in]
              n212 = in-place-cluster #9("Power Supply Object"=w471) -> (w455:T2)
            }
            n213 = property class="Mod Admin"(reference=w457) -> ("Accessors:Module ID"=w458:i32)  [unwired: 1 in, 2 out]
            n214 = Unbundle By Name(w464) -> ("Wait Notifier"=w463:refnum<notifier>, "wait for reply"=w462:bool)  [unwired: 1 out]
            n215 = Bundle By Name(cluster=T26 {"Module ID"=-1, "Volts"=0.0, "error"={"status"=FALSE, "code"=0, "source"=""}} ("read voltage (Reply Payload)"), "Module ID"=w458, "Volts"=w454, "error"=w453) -> (w461:T26)
            n216 = Merge Errors(w467, w453) -> (w459:errorcluster)
            n217 = case "DQMH_FIRE_NOTIFIER" shown="True" w462 {
              tunnel: w463 -> [_ w474]
              tunnel: w461 -> [_ w473]
              frame False {
              }
              frame True {
                n218 = Send Notification(notification=w473, notifier=w474) -> ()  [unwired: 1 in, 2 out]
              }
            }
          }
          frame "---Copy This Frame---" {
            # "Duplicate this frame when creating new messages.  Change this comment in the duplicated frame to describe this message."
            n219 = Merge Errors(w477) -> (w476:errorcluster)
          }
          frame "---Exit and Error Handling---" {
            # "Separator - the following cases handle errors and exit messages."
          }
          frame "Error" {
            # "#DQMH_CodeRecommended - If the module is running in standalone mode (External Launch = FALSE), this code will pop up an error dialog and call the 'Exit' message if an error occurs. Add more fine-grained error management here."
            # "Error - Check the error message data and respond accordingly. This message is sent by the \"Error Handler\" VIs at the end of each loop in this application."
            n220 = property on="Property Node" class="Mod Admin"(reference=w484) -> ("Accessors:External Launch"=w483:bool, "Accessors:Module ID"=w481:i32)  [unwired: 1 in, 2 out]
            n221 = Variant To Data(error in=w491, type=errorcluster {"status"=FALSE, "code"=0, "source"=""} ("error constant"), Variant=w485) -> (data=w480:errorcluster, error out=w489:errorcluster)
            n222 = local write "error out"(w480) -> ()
            n223 = call "Error Reported.vi"("Error"=w480, "Module ID"=w481) -> ()  [unwired: 9 in, 1 out]
            n224 = case shown="False" w483 {
              tunnel: [w496 _] -> w488
              tunnel: w482 -> [w494 _]
              tunnel: w480 -> [w495 _]
              frame False {
                n225 = disable-structure shown="Default" {
                  disable-tunnel: w495 -> [w497 _]
                  frame condition #0 (active) {
                    # "If the module is running standalone, then pop up an error dialog and call the \"Exit\" message."
                    n226 = call <vilib>:"Simple Error Handler.vi"("error in (no error)"=w497) -> ()  [unwired: 4 in, 5 out]
                  }
                  frame condition #1 {
                    # "To prevent the Simple Error Handler VI from being loaded (e.g. when deploying to a Real-Time target), add the Conditional Disable Symbol \"DQMH_Disable_SEH\" to your project and set it to TRUE."
                  }
                }
                n227 = call-poly <vilib>:"Delacor_lib_QMH_Enqueue Message (poly).vi"("Priority Message? (F)"=TRUE, "Message"="Exit", "Message Queue in"=w494) -> ("error out"=w496:errorcluster)  [unwired: 7 in, 1 out]
              }
              frame True {
                # "If the module was launched externally, calling the Error Reported broadcast VI is the only action performed by the \"Error\" message. The module's caller can then process the error appropriately."
              }
            }
            n228 = Merge Errors(w489, w488) -> (w487:errorcluster)
          }
          frame "Simulate MHL Error" {
            # "#DQMH_HowTo The 'Simulate MHL Error' button  illustrates how the MHL handles errors. This event is instructional in nature and can be removed."
            # "Simulate an error occurring at the MHL"
            n229 = property on="Property Node" class="Mod Admin"(reference=w503) -> ("Accessors:Module ID"=w504:i32)  [unwired: 1 in, 2 out]
            n230 = call "Module Name--constant.vi"("Module ID"=w504) -> ("Module Name"=w499:string)  [unwired: 10 in]
            n231 = Format Into String(format string="Simulated error originating at Message Handling Loop in %s", w499) -> (resulting string=w500:string)  [unwired: 2 in, 1 out]
            n232 = call <vilib>:"Error Cluster From Error Code.vi"("show call chain? (False)"=TRUE, "error message (\"\")"=w500, "error code (0)"=5001) -> ("error out"=w506:errorcluster)  [unwired: 6 in]
            n233 = Merge Errors(w508, w506) -> (w507:errorcluster)
          }
          frame "Exit" {
            w516 = 91  # 91: not all Exit messages will have an argument
            w517 = TRUE  # Stop the VI
            # "Release the message queue reference"
            # "#DQMH_CodeNeeded - Add any required cleanup code here."
            # "Exit - Exit the application."
            n234 = Variant To Data(error in=w525, type=T4 {"Module ID"=-1, "Origin"="", "Exit via Stop Module Req?"=FALSE, "Wait for Module to stop?"=FALSE} ("Stop Argument"), Variant=w515) -> (data=w512:T4, error out=w521:errorcluster)
            n235 = call <vilib>:"Clear Errors.vi"("error in (no error)"=w521, "specific error code to clear (0: all)"=w516) -> ("error out"=w524:errorcluster)  [unwired: 4 in, 1 out]
            n236 = property on="Property Node" class="Mod Admin"(reference=w510) -> ("Accessors:Module ID"=w509:i32)  [unwired: 1 in, 2 out]
            n237 = control-ref of="This VI"() -> (w511:refnum<vi>)
            n238 = call-dynamic "Delacor_lib_QMH_Release Message Queue.vi"("error in"=w524, "Message Queue"=w519) -> ("error out"=w523:errorcluster)  [unwired: 9 in]
            n239 = call "Handle Exit.vi"("Stop Argument"=w512, "Module Admin in"=w510, "VI reference"=w511) -> ("error out"=w522:errorcluster, "Wait for Stop?"=w513:bool)  [unwired: 7 in]
            n240 = Merge Errors(w523, w522) -> (w520:errorcluster)
            n241 = call "Error Reported.vi"("Error"=w520, "Module ID"=w509) -> ()  [unwired: 9 in, 1 out]
          }
          frame Default {
            # "'Default' case only runs if there is a message that isn't defined in any of the other cases.  Output a programming error."
            n242 = property on="Property Node" class="Mod Admin"(reference=w533) -> ("Accessors:Module ID"=w532:i32)  [unwired: 1 in, 2 out]
            n243 = call "Module Name--constant.vi"("Module ID"=w532) -> ("Module Name"=w526:string)  [unwired: 10 in]
            n244 = Format Into String(format string="The invalid message string \"%s\" was received in the Message Handling Loop for module \"%s\".", w527, w526) -> (resulting string=w529:string)  [unwired: 2 in, 1 out]
            n245 = call <vilib>:"Error Cluster From Error Code.vi"("show call chain? (False)"=TRUE, "error message (\"\")"=w529, "error code (0)"=1) -> ("error out"=w535:errorcluster)  [unwired: 6 in]
            n246 = Merge Errors(w536, w535) -> (w537:errorcluster)
          }
        }
        n247 = call-dynamic "Delacor_lib_QMH_Error Handler - Message Handling Loop.vi"("error in"=w254, "Message Queue in"=w245) -> ("dup error in"=w251:errorcluster)  [unwired: 8 in, 1 out]
      }
    }
    frame Error {
      n248 = call "Synchronize Caller Events.vi"("Module Admin"=w541) -> ("Module Admin out"=w540:refnum<class "Delacor_lib_QMH_Cloneable Module Admin.lvclass">)  [unwired: 9 in, 1 out]
      n249 = property on="Property Node" class="Mod Admin"(reference=w540) -> ("Accessors:Module ID"=w539:i32)  [unwired: 1 in, 2 out]
      n250 = call-dynamic "Delacor_lib_QMH_Release Message Queue.vi"("error in"=w547, "Message Queue"=w538) -> ("error out"=w546:errorcluster)  [unwired: 9 in]
      n251 = call "Module Name--constant.vi"("Module ID"=w539) -> ("Module Name"=w544:string)  [unwired: 10 in]
      n252 = Format Into String(format string="An error occurred during initialization. %s is no longer running.", w544) -> (resulting string=w542:string)  [unwired: 2 in, 1 out]
      n253 = call "Error Reported.vi"("Additional Information"=w542, "Error"=w546, "Module ID"=w539) -> ()  [unwired: 8 in, 1 out]
    }
  }
  n254 = Merge Errors(w17, w16) -> (w18:errorcluster)
  n255 = call "Close Module.vi"("error in"=w18, "Wait for stop?"=w2, "Module Admin in"=w4) -> ("error out"=w14:errorcluster, "External Launch"=w1:bool, "Module Admin out"=w3:refnum<class "Delacor_lib_QMH_Cloneable Module Admin.lvclass">)  [unwired: 6 in]
  n256 = Unregister For Events(event registration refnum=w9, error in=w14) -> (error out=w13:errorcluster)
  "error out" <- w13
  n257 = case "External Launch?" shown="True" w1 {
    tunnel: w13 -> [_ w548]
    frame False {
    }
    frame True {
      n258 = case shown="No Error" w548 {
        frame No Error {
          n259 = invoke class="VI" method="FP.Close"() -> ()  [unwired: 3 in, 3 out]
        }
        frame Error {
          n260 = disable-structure shown="Default" {
            frame condition #0 (active) {
              n261 = invoke class="VI" method="FP.Open"("Activate"=TRUE ("Activate?")) -> ()  [unwired: 4 in, 5 out]
            }
            frame condition #1 {
              # "Don't show panel on error if running inside a built EXE."
            }
          }
        }
      }
    }
  }
  n262 = local write "Module Admin"(w3) -> ()
